vi "load waveforms_tt2.vi"(1 "waveform":path) -> (0 "# of points":i32)   [LabVIEW 2010]
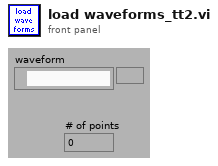
[diagram p1: front panel]
types:
  T1 = cluster{"Xpixels":i32, "Vx-min ref":dbl, "Vx-max ref":dbl, "Ypixels":i32, "Vy-min ref":dbl, "Vy-max ref":dbl, "srate":dbl, "type":string, "date":string, "time":string, "Colormap":u16, "square pixels":bool, "square matrix":bool, "Xpixels Img":i32, "Vx-min Img":dbl, "VX-max Img":dbl, "Ypixels Img":i32, "Vy-min Img":dbl, "Vy-max Img ":dbl, "autoshutter":bool, "P":dbl, "sAOxy":i32, "finite":bool, "cont":bool, "wavdet":bool, "measpoints":i32, "avpp":i32, "bufferAO":i32, "bufferAI":i32, "CH1":bool, "CH2":bool, "X":bool, "Y":bool, "timeout":dbl, "starttick":u32, "waveform":path, "Vy-ref":dbl, "Vx-ref":dbl, "refreshrate":dbl}
  T2 = cluster{"VtoP":dbl[], "CWlasers":dbl[], "shutter":dbl[]}
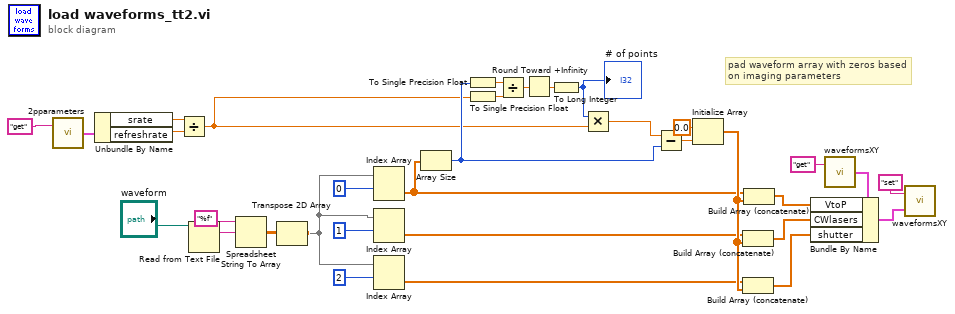
[diagram p0: block diagram]
diagram:
  # "pad waveform array with zeros based\non imaging parameters"
  n1 = call "2pparameters.vi"("command"="get") -> ("Params out"=w12:T1)  [unwired: 1 in]
  n2 = Unbundle By Name(w12) -> ("srate"=w33:dbl, "refreshrate"=w31:dbl)
  n3 = Divide(x=w33, y=w31) -> (x/y=w2:dbl)
  n4 = Read from Text File(file (use dialog)="waveform") -> (text=w10:string)  [unwired: 3 in, 3 out]
  n5 = Spreadsheet String To Array(format string="%f", spreadsheet string=w10) -> (array=w8:dbl[][])  [unwired: 2 in]
  n6 = Transpose 2D Array(2D array=w8) -> (transposed array=w4:dbl[][])
  n7 = Index Array(array=w4, index (row)=0) -> (element=w23:dbl[])  [unwired: 1 in]
  n8 = Index Array(array=w4, index (row)=1) -> (element=w24:dbl[])  [unwired: 1 in]
  n9 = Index Array(array=w4, index (row)=2) -> (element=w25:dbl[])  [unwired: 1 in]
  n10 = Array Size(array=w23) -> (size(s)=w3:i32)
  n11 = To Single Precision Float(number=w3) -> (single precision float=w13:sgl)
  n12 = To Single Precision Float(number=w2) -> (single precision float=w14:sgl)
  n13 = Divide(x=w13, y=w14) -> (x/y=w15:sgl)
  n14 = Round Toward +Infinity(x=w15) -> (ceil(x): smallest int >= x=w16:sgl)
  n15 = To Long Integer(number=w16) -> (32bit integer=w30:i32)
  "# of points" <- w30
  n16 = Multiply(x=w30, y=w2) -> (x*y=w32:dbl)
  n17 = Subtract(x=w32, y=w3) -> (x-y=w21:dbl)
  n18 = Initialize Array(0.0 ("element"), w21) -> (w26:dbl[])
  n19 = Build Array (concatenate)(w24, w26) -> (w28:dbl[])
  n20 = Build Array (concatenate)(w25, w26) -> (w29:dbl[])
  n21 = Build Array (concatenate)(w23, w26) -> (w27:dbl[])
  n22 = call "waveformsXY.vi"("command"="get") -> ("waveforms out"=w18:T2)  [unwired: 1 in]
  n23 = Bundle By Name(cluster=w18, "VtoP"=w27, "CWlasers"=w28, "shutter"=w29) -> (w20:T2)
  n24 = call "waveformsXY.vi"("waveforms in"=w20, "command"="set") -> ()  [unwired: 1 out]
